vi "To JSON.vi"(8 "error in":errorcluster, 10 "JSON Config":path, 11 "object in":refnum<class "Camera Imaqdx CFG.lvclass">) -> (0 "error out":errorcluster, 3 "object out":refnum<class "Camera Imaqdx CFG.lvclass">)   [LabVIEW 2023, in "Camera Imaqdx CFG.lvclass"]
uses:
  Camera Imaqdx CFG.lvclass
  Camera Imaqdx CFG.lvclass/Camera Imaqdx CFG.ctl
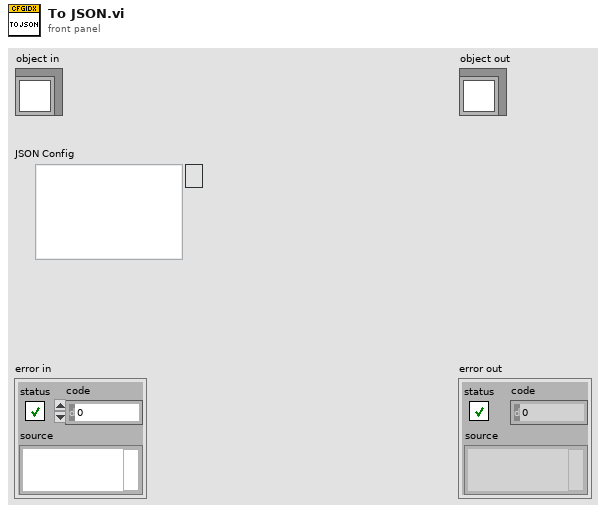
[diagram p1: front panel]
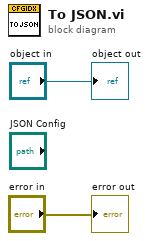
[diagram p0: block diagram]
diagram:
  "error out" <- "error in"
  "object out" <- "object in"
